vi "Reserve Sessions.vi"(6 "timeout (ms)":i32, 8 "error in":errorcluster, 9 "instrument type id":string, 10 "pin or relay names":string[](array[string]), 11 "pin map context":T1) -> (0 "error out":errorcluster, 3 "session reservation out":refnum<class "Session Reservation.lvclass">)   [LabVIEW 2020, in "MeasurementLink Session Management V1.lvlib" / "Session Reservation.lvclass"]
doc: "Reserves session(s) based on the provided instrument type and pin information."
uses:
  Session Reservation.lvclass
  MeasurementLink Session Management Client/RPC Messages/ni_measurementlink_PinMapContext.ctl
  IReservationObserver/IReservationObserver.lvclass
  MeasurementLink Session Management Client/MeasurementLink Session Management Client.lvlib
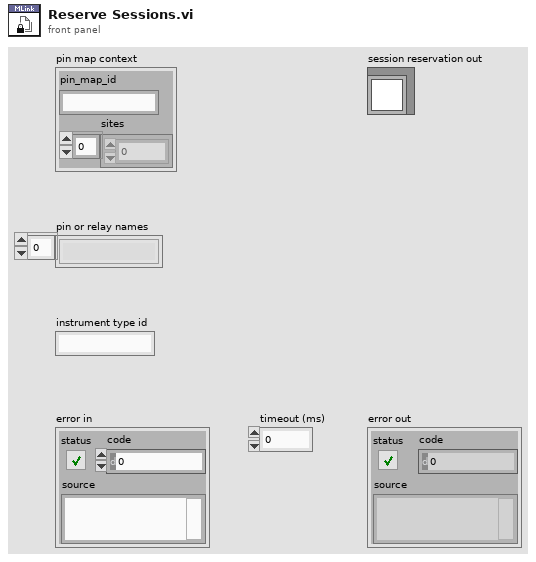
[diagram p1: front panel]
types:
  T1 = typedef "MeasurementLink Session Management Client.lvlib/ni_measurementlink_PinMapContext.ctl" = cluster{"pin_map_id":string, "sites":i32[]}
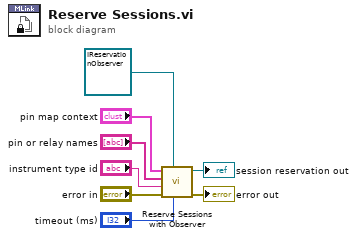
[diagram p0: block diagram]
diagram:
  n1 = call "Reserve Sessions with Observer.vi"("timeout (ms)"="timeout (ms)", "reservation observer"=refnum<class "IReservationObserver.lvclass"> refnum, "error in"="error in", "instrument type id"="instrument type id", "pin or relay names"="pin or relay names", "pin map context"="pin map context") -> ("error out"=→"error out":errorcluster, "session reservation out"=→"session reservation out":refnum<class "Session Reservation.lvclass">)  [unwired: 4 in]
